vi "Symmetrical Components.vi"(0 "voltage spectra":T2(array[cluster]), 5 "current spectra":T2(array[cluster]), 9 "system info in":refnum<class "EP System Info.lvclass">, 11 "error in (no error)":errorcluster) -> (4 "symmetrical components":T4, 6 "power symmetrical components":T3, 10 "system info out":refnum<class "EP System Info.lvclass">, 15 "error out":errorcluster)   [LabVIEW 2014, in "NI_EP_Power Quality.lvlib"]
doc: "Calculates voltage, current, and power symmetrical components for a 10-cycle or 12-cycle block. Use the results of this VI to analyze the voltage or current unbalance of a three-phase electrical power system.\n\nThis VI supports measuring single-line and multiple-line systems."
uses:
  <vilib>/addons/Electrical Power/PQ/NI_EP_Power Quality.lvlib
  <vilib>/addons/Electrical Power/PQ/Common/Controls/ep_AI Data Channel.ctl
  <vilib>/addons/Electrical Power/PQ/Common/Classes/System Info/EP System Info.lvclass
  <vilib>/addons/Electrical Power/Motor Monitoring/NI_EP_Motor Monitoring.lvlib
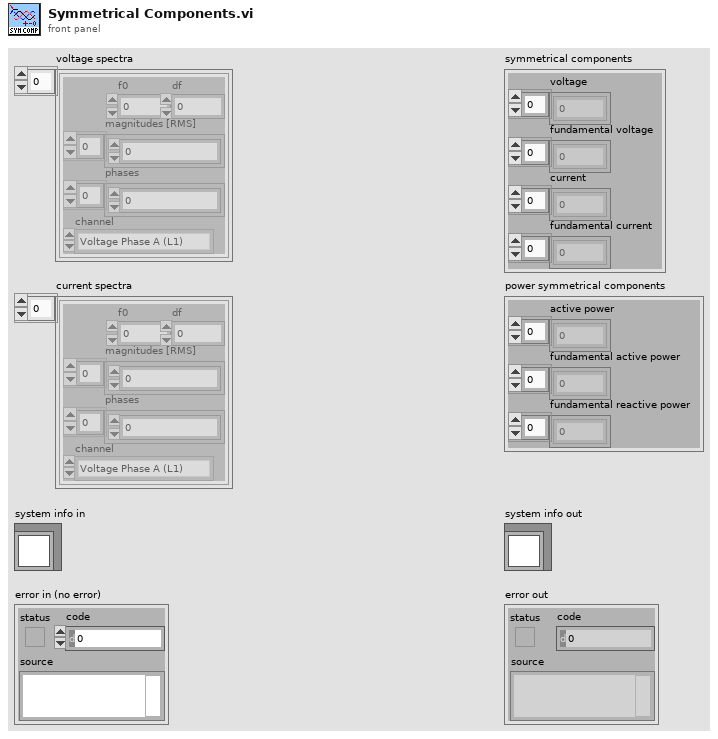
[diagram p1: front panel]
types:
  T1 = typedef "NI_EP_Power Quality.lvlib/ep_AI Data Channel.ctl" = enum16{"Voltage Phase A (L1)", "Voltage Phase B (L2)", "Voltage Phase C (L3)", "Voltage Phase N (Neutral)", "Current Phase A (L1)", "Current Phase B (L2)", "Current Phase C (L3)", "Current Phase N (Neutral)"}
  T2 = cluster{"f0":dbl, "df":dbl, "magnitudes [RMS]":dbl[], "phases":dbl[], "channel":T1}[]
  T3 = cluster{"active power":dbl[], "fundamental active power":dbl[], "fundamental reactive power":dbl[]}
  T4 = cluster{"voltage":dbl[], "fundamental voltage":dbl[], "current":dbl[], "fundamental current":dbl[]}
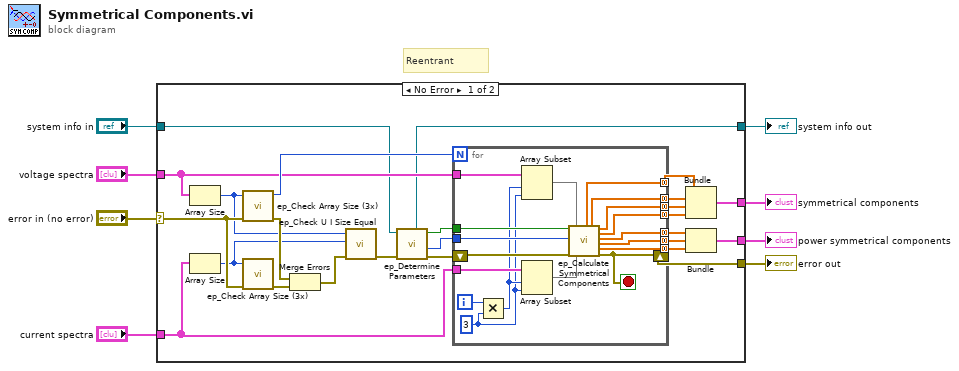
[diagram p0: block diagram]
diagram:
  # "Reentrant"
  n1 = case shown="No Error" "error in (no error)" {
    selector: "error in (no error)" -> [w27 w53]
    tunnel: "system info in" -> [w14 w52]
    tunnel: "voltage spectra" -> [w15 _]
    tunnel: "current spectra" -> [w17 _]
    tunnel: [w31 _] -> w5
    tunnel: [w30 _] -> w1
    tunnel: [w13 w52] -> w4
    tunnel: [w29 w53] -> w3
    frame No Error {
      n2 = Array Size(array=w15) -> (size(s)=w10:i32)
      n3 = Array Size(array=w17) -> (size(s)=w9:i32)
      n4 = call <vilib>:"ep_Check Array Size (3x).vi"("error in (no error)"=w27, "number of channels"=w10) -> ("error out"=w26:errorcluster, "number of 3 phases"=w16:i32)  [unwired: 8 in]
      n5 = call <vilib>:"ep_Check Array Size (3x).vi"("error in (no error)"=w27, "number of channels"=w9) -> ("error out"=w25:errorcluster)  [unwired: 8 in, 1 out]
      n6 = Merge Errors(w26, w25) -> (w11:errorcluster)
      n7 = call <vilib>:"ep_Check U I Size Equal.vi"("error in (no error)"=w11, "current channel number"=w9, "voltage channel number"=w10) -> ("error out"=w12:errorcluster)  [unwired: 8 in]
      n8 = call <vilib>:"ep_Determine Parameters.vi"("error in (no error)"=w12, "system info in"=w14) -> ("error out"=w28:errorcluster, "cycles per block"=w32:i32, "line voltage?"=w33:bool, "system info out"=w13:refnum<class "EP System Info.lvclass">)  [unwired: 6 in]
      n9 = for {
        N: w16 -> [_]
        tunnel: w33 -> [w49]
        shift-right: [w50] -> w29
        shift-left: w28 -> [w51]
        tunnel: w32 -> [w48]
        tunnel: w15 -> [w37]
        tunnel: [w47] -> w24 mode=concatenating
        tunnel: [w46] -> w23 mode=concatenating
        tunnel: [w45] -> w22 mode=concatenating
        tunnel: [w44] -> w21 mode=concatenating
        tunnel: [w43] -> w20 mode=concatenating
        tunnel: [w42] -> w19 mode=concatenating
        tunnel: [w41] -> w18 mode=concatenating
        tunnel: w17 -> [w40]
        i -> [w39]
        stop <- w50 stop-if-true
        w35 = 3 ("x")
        n10 = Multiply(x=w39, y=w35) -> (x*y=w36:i32)
        n11 = Array Subset(array=w37, index=w36, length=w35) -> (w34:T2)
        n12 = Array Subset(array=w40, index=w36, length=w35) -> (w38:T2)
        n13 = call <vilib>:"ep_Calculate Symmetrical Components.vi"("line voltage? (F)"=w49, "cycles per block"=w48, "error in (no error)"=w51, "voltage complex spectra (5Hz step)"=w34, "current complex spectra (5Hz step)"=w38) -> ("voltage"=w47:dbl[], "fundamental voltage"=w46:dbl[], "current"=w45:dbl[], "fundamental current"=w44:dbl[], "active power"=w43:dbl[], "fundamental active power"=w42:dbl[], "fundamental reactive power"=w41:dbl[], "error out"=w50:errorcluster)  [unwired: 7 in]
      }
      n14 = Bundle("voltage"=w24, "fundamental voltage"=w23, "current"=w22, "fundamental current"=w21) -> (w31:T4)  [unwired: 1 in]
      n15 = Bundle("active power"=w20, "fundamental active power"=w19, "fundamental reactive power"=w18) -> (w30:T3)  [unwired: 1 in]
    }
    frame Error {
    }
  }
  "error out" <- w3
  "symmetrical components" <- w5
  "power symmetrical components" <- w1
  "system info out" <- w4
